vi "Create_copy_of_pdf in day folder.vi"(1 "Top Level":bool, 2 "Path name Out":path) -> ()   [LabVIEW 2015]
panel:
  out "Copy from this file":path
  out "replace this file":path
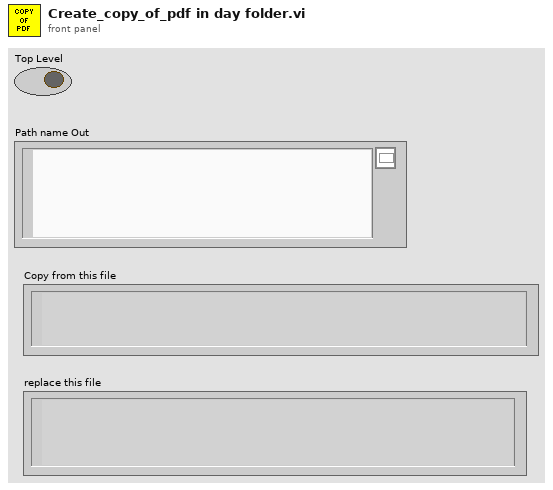
[diagram p1: front panel]
types:
  T1 = typedef "LVDateTimeRec.ctl" = cluster{"fractional second":dbl, "second":i32, "minute":i32, "hour":i32, "day of month":i32, "month":i32, "year":i32, "day of week":i32, "day of year":i32, "DST":i32}
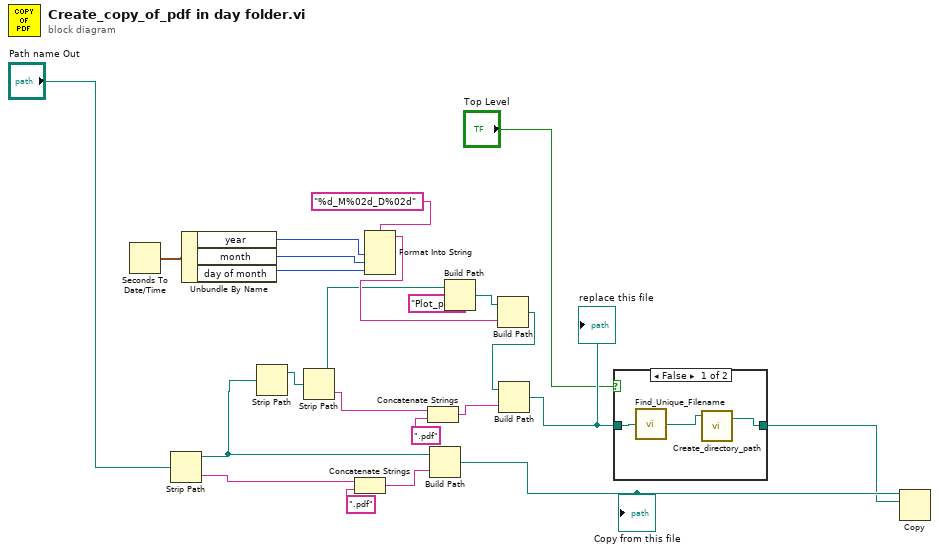
[diagram p0: block diagram]
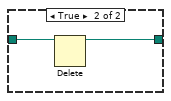
[diagram p2: hidden frame]
diagram:
  n1 = Seconds To Date/Time() -> (date time rec=w22:T1)  [unwired: 2 in]
  n2 = Strip Path(path="Path name Out") -> (stripped path=w5:path, name=w2:string)
  n3 = Unbundle By Name(w22) -> ("year"=w21:i32, "month"=w20:i32, "day of month"=w19:i32)
  n4 = Strip Path(path=w5) -> (stripped path=w9:path)  [unwired: 1 out]
  n5 = Strip Path(path=w9) -> (stripped path=w12:path, name=w10:string)
  n6 = Concatenate Strings(w2, ".pdf" ("string")) -> (w4:string)
  n7 = Format Into String(format string="%d_M%02d_D%02d", w21, w20, w19) -> (resulting string=w23:string)  [unwired: 2 in, 1 out]
  n8 = Concatenate Strings(w10, ".pdf" ("string")) -> (w15:string)
  n9 = Build Path(base path=w5, name or relative path=w4) -> (appended path=w8:path)
  "Copy from this file" <- w8
  n10 = Build Path(base path=w12, name or relative path="Plot_pdfs") -> (appended path=w14:path)
  n11 = Build Path(base path=w14, name or relative path=w23) -> (appended path=w16:path)
  n12 = Build Path(base path=w16, name or relative path=w15) -> (appended path=w17:path)
  "replace this file" <- w17
  n13 = case shown="False" "Top Level" {
    tunnel: w17 -> [w26 w28]
    tunnel: [w24 w27] -> w6
    frame False {
      n14 = call "Find_Unique_Filename.vi"("Path In"=w26) -> ("Unique Path Out"=w25:path)  [unwired: 2 in]
      n15 = call "Create_directory_path.vi"("Path name"=w25) -> ("Path name Out"=w24:path)  [unwired: 2 in, 1 out]
    }
    frame True {
      n16 = Delete(path (use dialog)=w28) -> (deleted path=w27:path)  [unwired: 4 in, 2 out]
    }
  }
  n17 = Copy(10:w6, 11:w8) -> ()  [unwired: 3 in, 3 out]
